vi "UI-电源头正面标签3检测.vi"(8 "error in (no error)":errorcluster caption="错误输入（无错误）", 11 "名称或相对路径":string="Template Program") -> (0 "error in (no error) 2":errorcluster caption="错误输入（无错误）")   [LabVIEW 2017]
uses:
  Global System.vi
  <vilib>/Utility/xml.llb/Write to XML File(string).vi
  Picture/SaveButtom.ctl
panel:
  in  "获取图像":bool
  in  "ROI获取":bool
  in  "创建模板":bool
  in  "保存图像":bool
  out "添加的路径":path
  in  "刷新":bool
  in  "测试按钮":bool
  in  "保存按钮":bool
  in  "Main":enum32{"主参数", "模板匹配参数 ", "测试效果"}(tab)
  in  "UI电源线正面标签3基础参数":T1={"IsNorImage"=TRUE, "Exposure Values"=100289, "ImagePath"=path "C:/Users/hedongpo/Desktop/514-hdp/Alignment Assemble System/Test Picture/B/3.bmp"} caption="参数界面" {"Exposure Values" scale=0.0..200000.0}
  in  "UI电源线正面标签3参数":T3={"Rectangle"={"Left"=0, "Top"=0, "Right"=0, "Bottom"=0, "Rotation"=0.0}, "Algorithm "=2, "Parameters"={"Number of Matches Requested"=1, "Minimum Match Score"=800.0, "Angle Ranges"=[{"Start Angle"=-180.0, "End Angle"=180.0}]}, "Advanced Options "=[{"Item"=102, "Value"=10.0}, {"Item"=106, "Value"=300.0}, {"Item"=107, "Value"=0.0}, {"Item"=108, "Value"=6.0}, {"Item"=109, "Value"=1.0}, {"Item"=114, "Value"=25.0}, {"Item"=111, "Value"=20.0}, {"Item"=112, "Value"=10.0}, {"Item"=113, "Value"=20.0}, {"Item"=103, "Value"=1.0}, {"Item"=104, "Value"=20.0}, {"Item"=105, "Value"=0.0}, {"Item"=100, "Value"=5.0}], "模板路径"=path "", "Color Plane "=0} {"Color Plane" items=["Red", "Green", "Blue", "Hue", "Saturation", "Luminance", "Value", "Intensity"]; "Advanced Options"."Item" items=["LD Sampling - Minimum Constrast"=0, "LD Sampling - Enable Subpixel Accuracy"=1, "LD Sampling - Search Strategy"=2, "LD Sampling - Subpixel Iterations"=3, "LD Sampling - Subpixel Tolerance"=4, "LD Sampling - Initial Match List Length"=5, "LD Sampling - Match List Reduction Factor"=6, "LD Sampling - Initial Step Size"=7, "LD Sampling - Intermediate Angular Accuracy"=8, "-"=9, "Pyramid - Max Pyramid Level"=100, "Pyramid - Minimum Contrast"=102, "Pyramid - Enable Subpixel Accuracy"=103, "Pyramid - Subpixel Iterations"=104, "Pyramid - Subpixel Tolerance"=105, "Pyramid - Initial Match List Length"=106, "Pyramid - Match List Reduction Factor"=107, "Pyramid - Intermediate Angular Accuracy"=108, "Pyramid - Process Border Matches"=109, "Pyramid - Min Match Separation Distance"=111, "Pyramid - Min Match Separation Angle"=112, "Pyramid - Max Match Overlap"=113, "Pyramid - Max Cache in MB"=114, "Pyramid - Clear Cache"=115, "-"=116, "Enable Defect Map"=200]; "Algorithm" items=["All", "Low Discrepancy Sampling", "Grayscale Value Pyramid", "Gradients Pyramid"]; "Rectangle"."Rotation" format="%.2f"; "Rectangle"."Left" scale=0.0..1024.0; "Rectangle"."Right" scale=0.0..1024.0}
  out "结果":bool
  out "原始图像":T4(plugin-control)
  out "模板图片":T4(plugin-control)
  out "路径输出":path
  in  "Vision Paramter Save Buttom":T5
  out "system time":string
  in  "取消按钮":bool
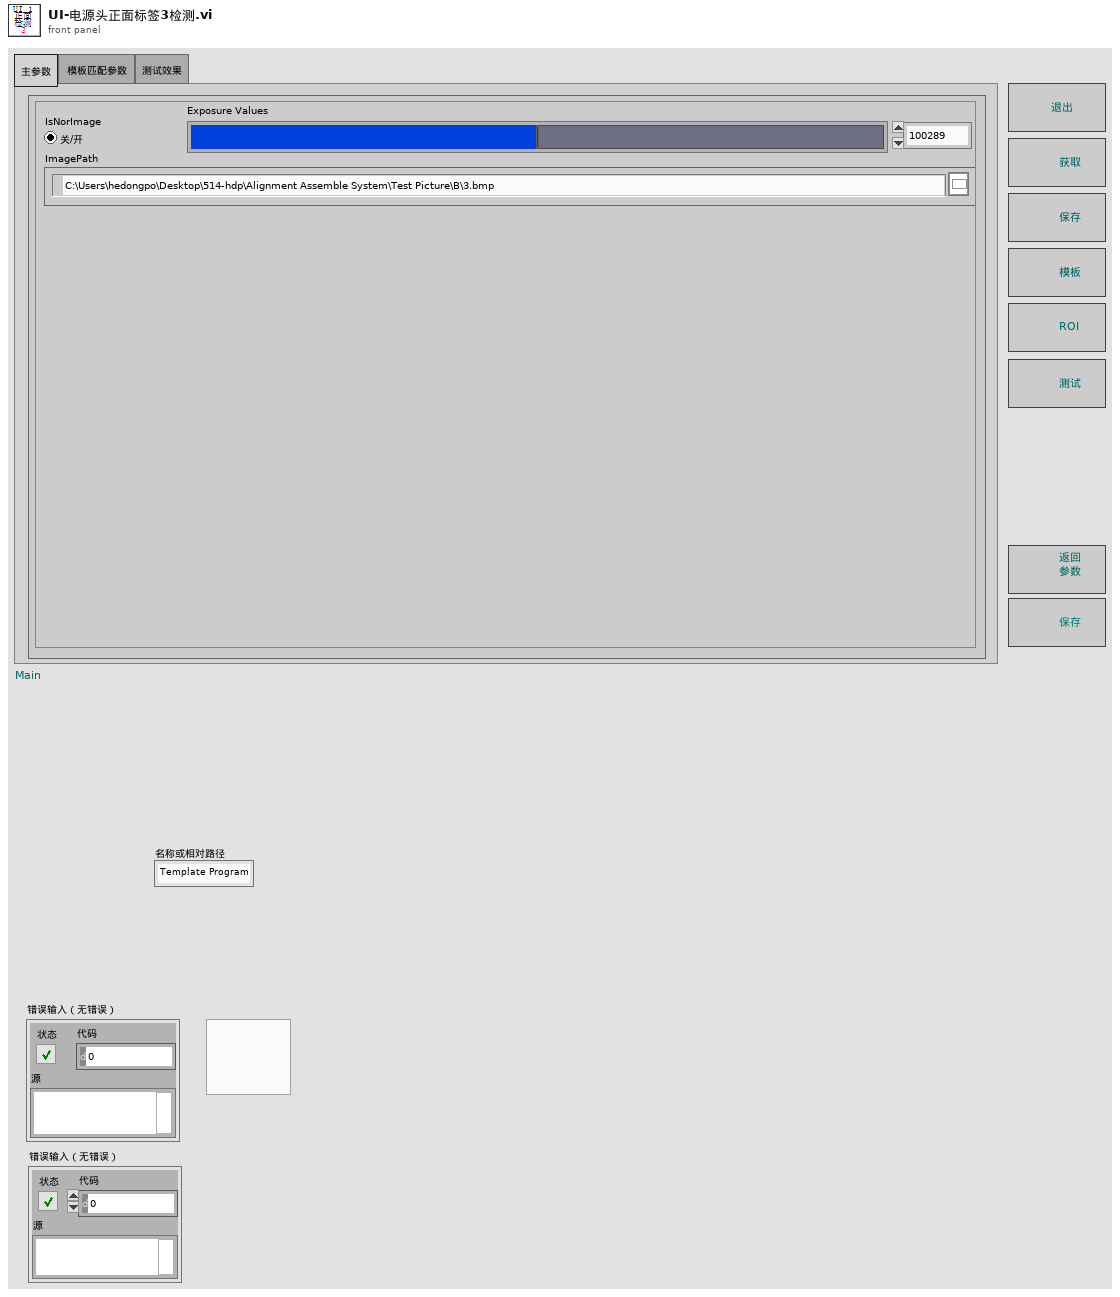
[diagram p1: front panel]
types:
  T1 = cluster{"IsNorImage":bool, "Exposure Values":u32, "ImagePath":path}
  T2 = typedef "IMAQ Rectangle" = cluster{"Left":i32, "Top":i32, "Right":i32, "Bottom":i32, "Rotation":dbl}
  T3 = cluster{"Rectangle":T2, "Algorithm ":i32, "Parameters":cluster{"Number of Matches Requested":i32, "Minimum Match Score":sgl, "Angle Ranges":cluster{"Start Angle":sgl, "End Angle":sgl}[]}, "Advanced Options ":cluster{"Item":u16, "Value":dbl}[], "模板路径":path, "Color Plane ":i32}
  T4 = typedef "IMAQ Image.ctl" = refnum<image>
  T5 = typedef "SaveButtom.ctl" = bool
  T6 = cluster{"index":i32, "this vi":refnum<vi>, "error out":errorcluster}
  T7 = cluster{"master data":string, "priority":u16, "secondary data":string[]}
  T8 = cluster{"case name":string[], "queue array":refnum<queue>[]}
  T9 = typedef "Image Type" = u32
  T10 = cluster{"Global Rectangle":i32[], "Contours":cluster{"Contour Type":u32, "ROI Type":u32, "Points":i32[]}[]}
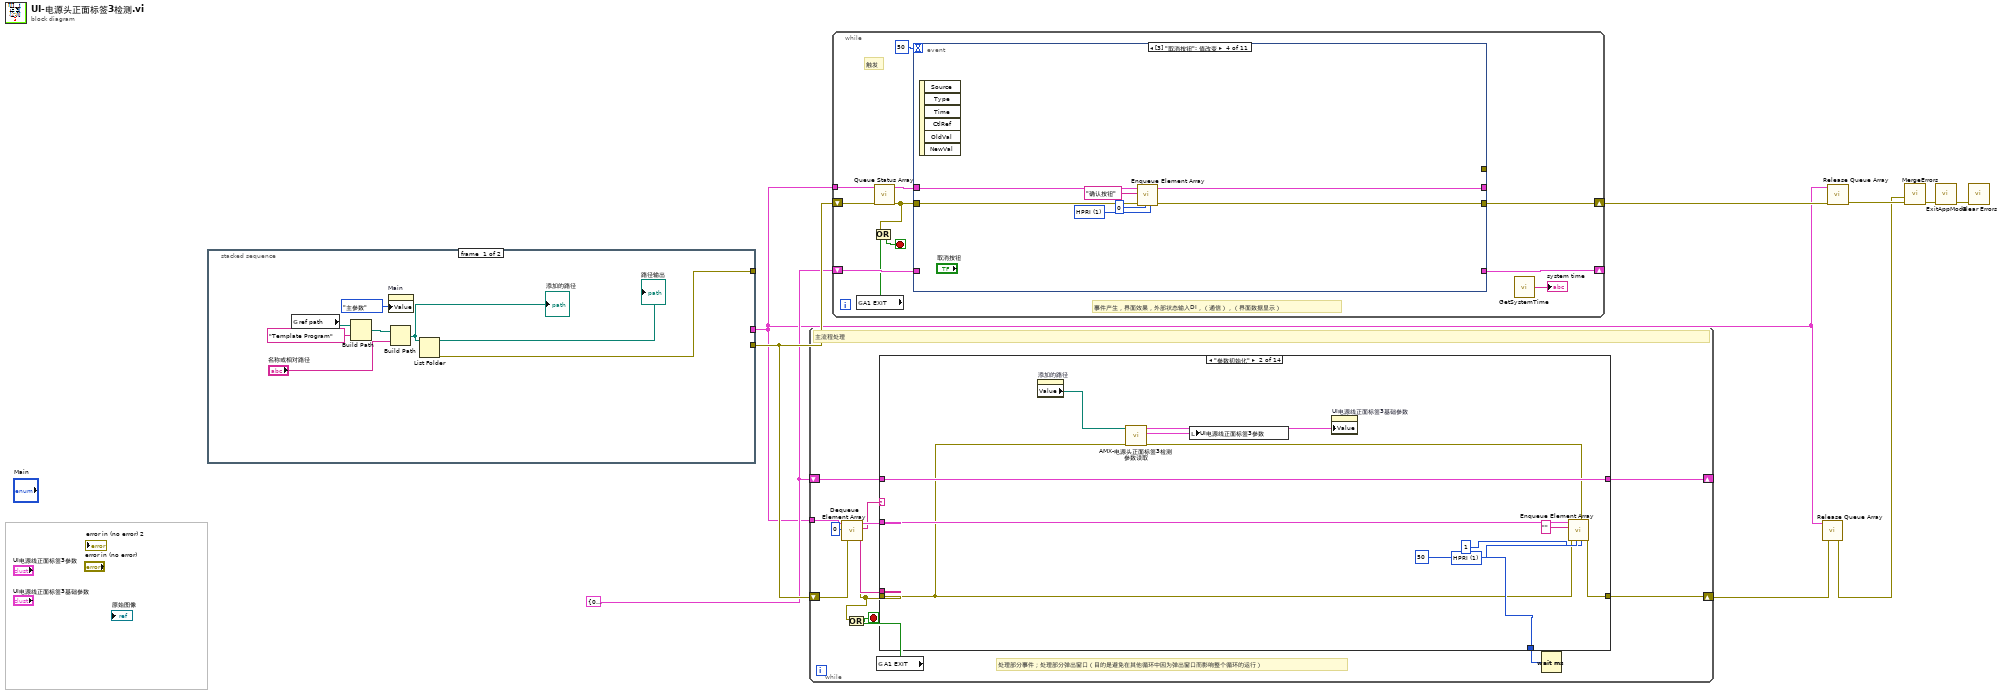
[diagram p0: block diagram]
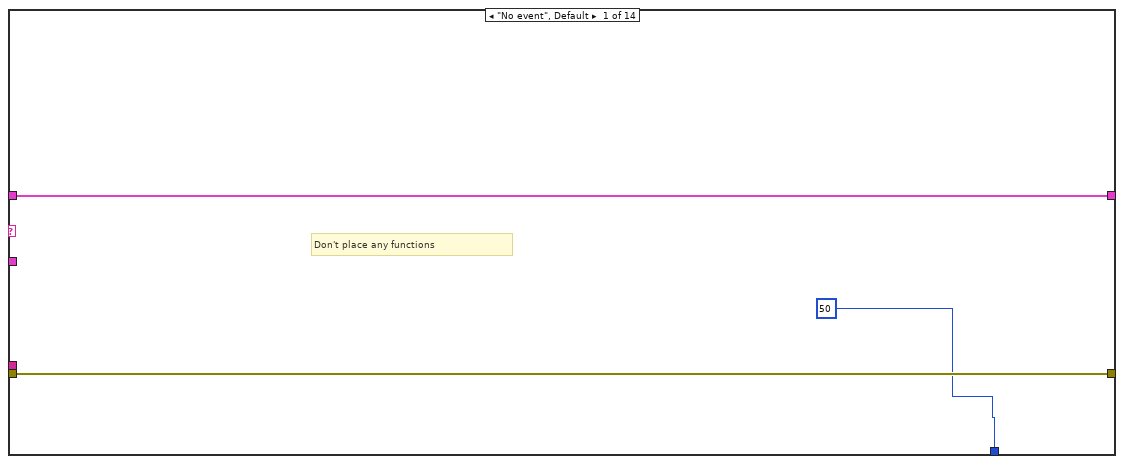
[diagram p2: hidden frame]
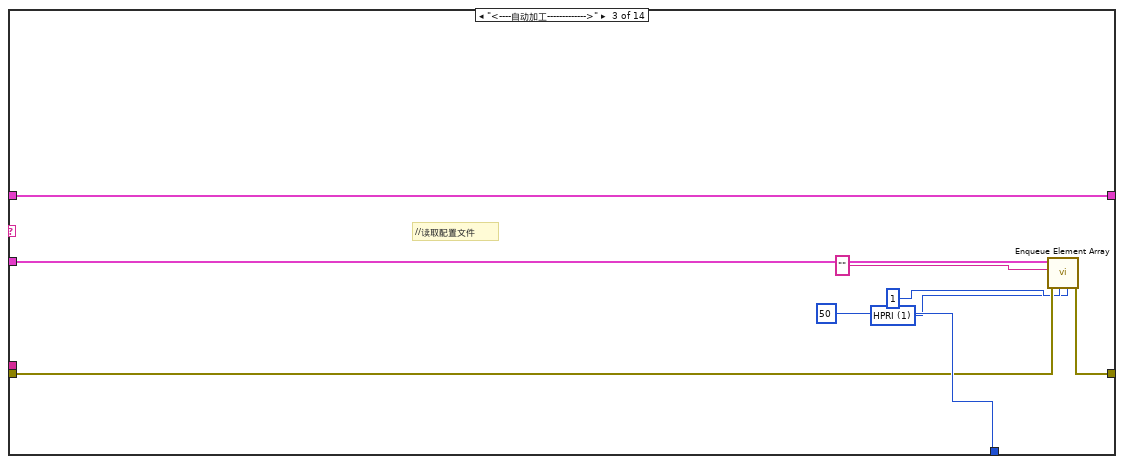
[diagram p3: hidden frame]
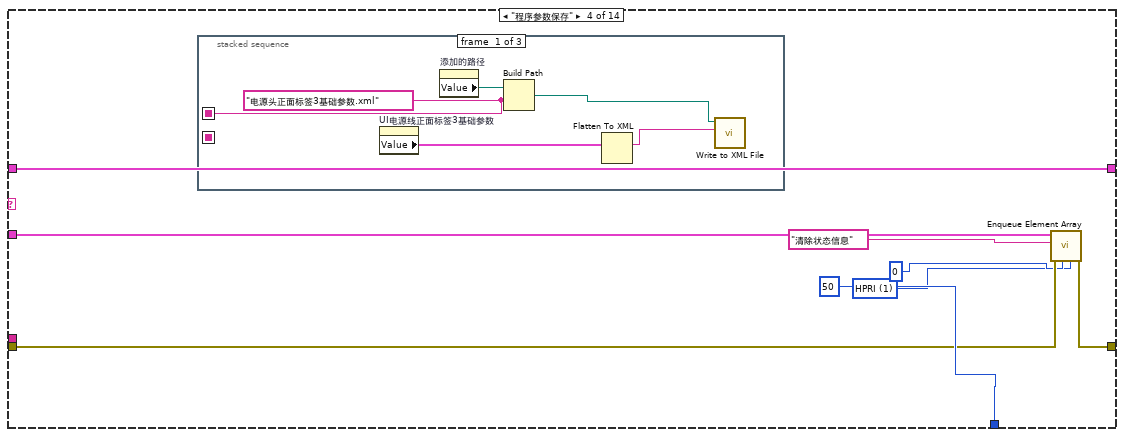
[diagram p4: hidden frame]
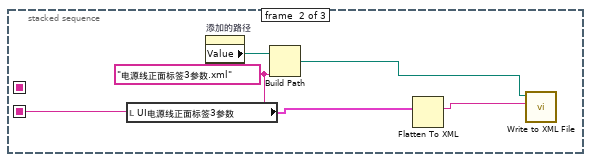
[diagram p5: hidden frame]
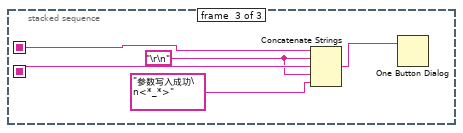
[diagram p6: hidden frame]
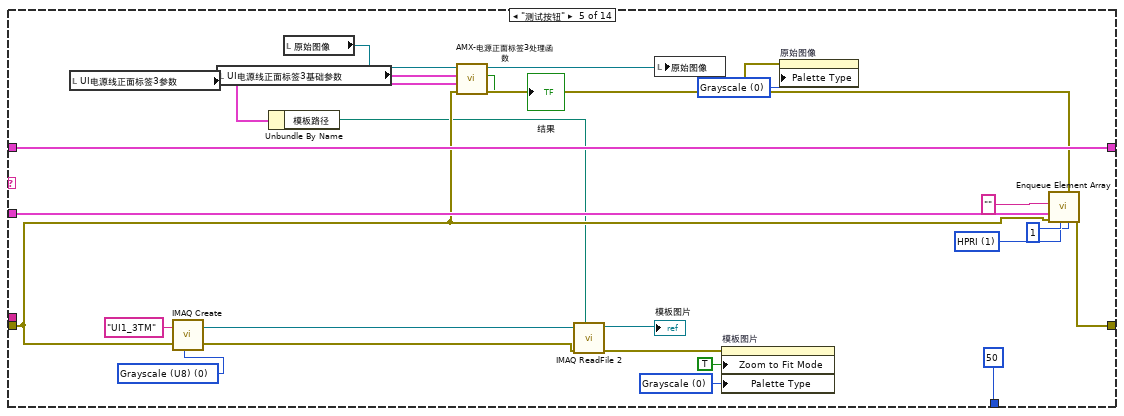
[diagram p7: hidden frame]
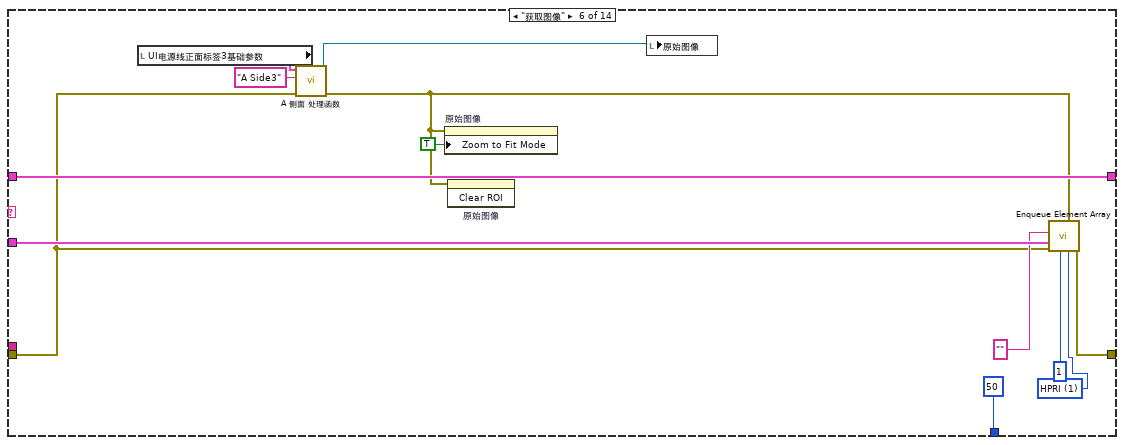
[diagram p8: hidden frame]
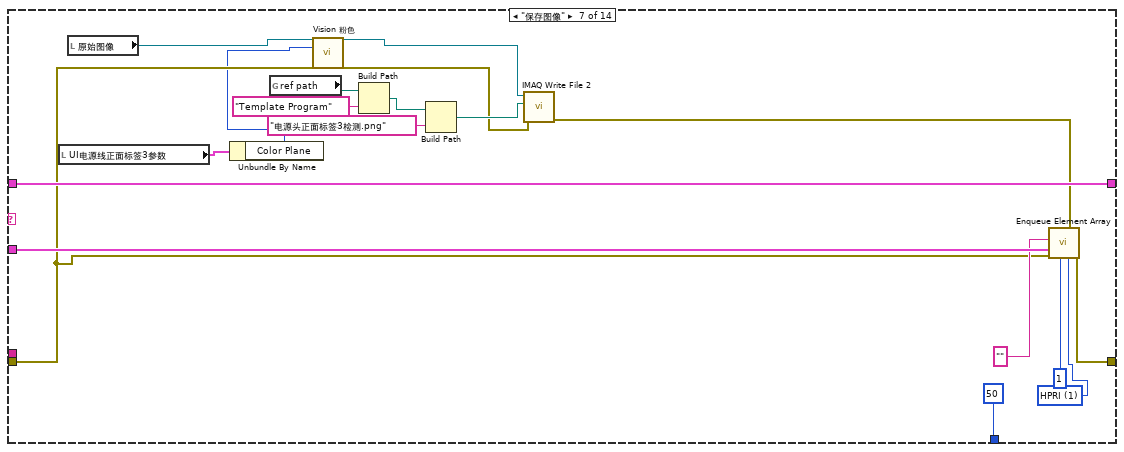
[diagram p9: hidden frame]
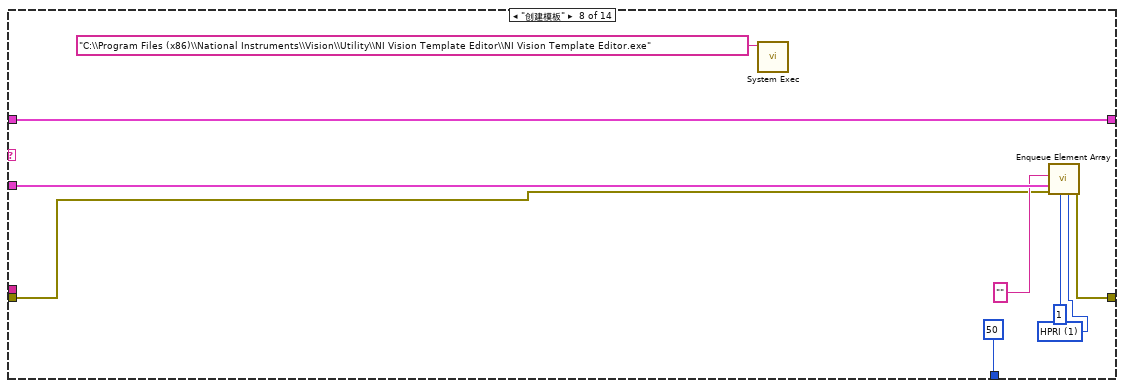
[diagram p10: hidden frame]
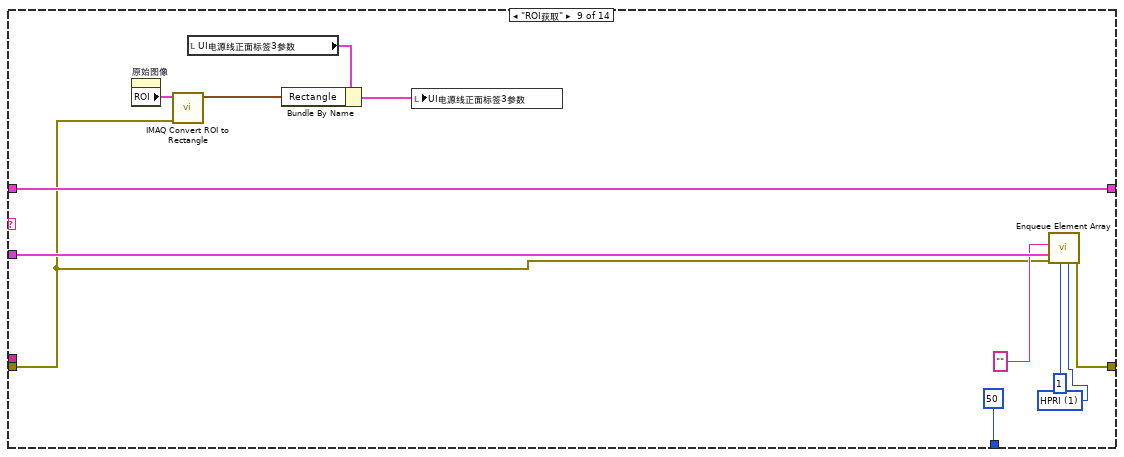
[diagram p11: hidden frame]
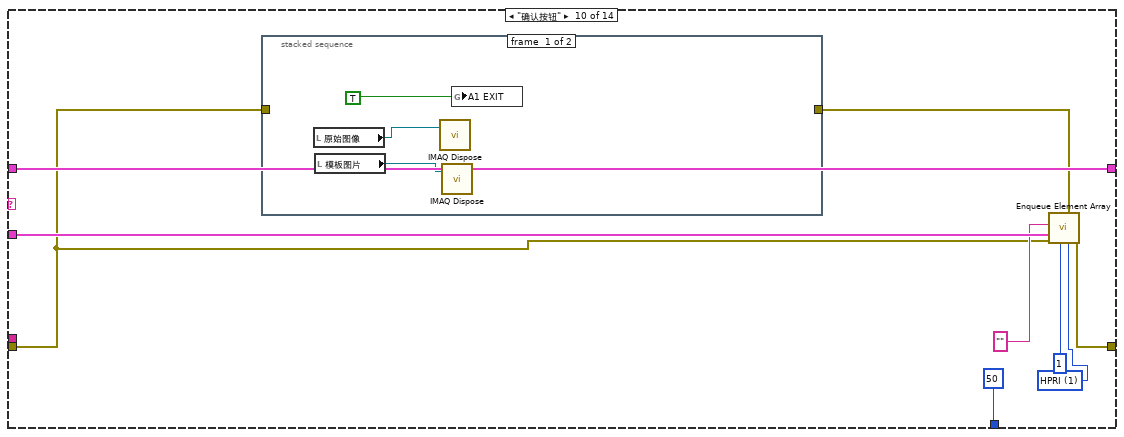
[diagram p12: hidden frame]
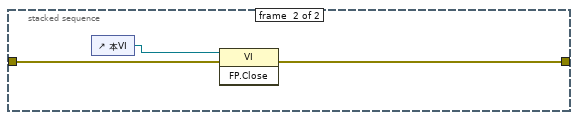
[diagram p13: hidden frame]
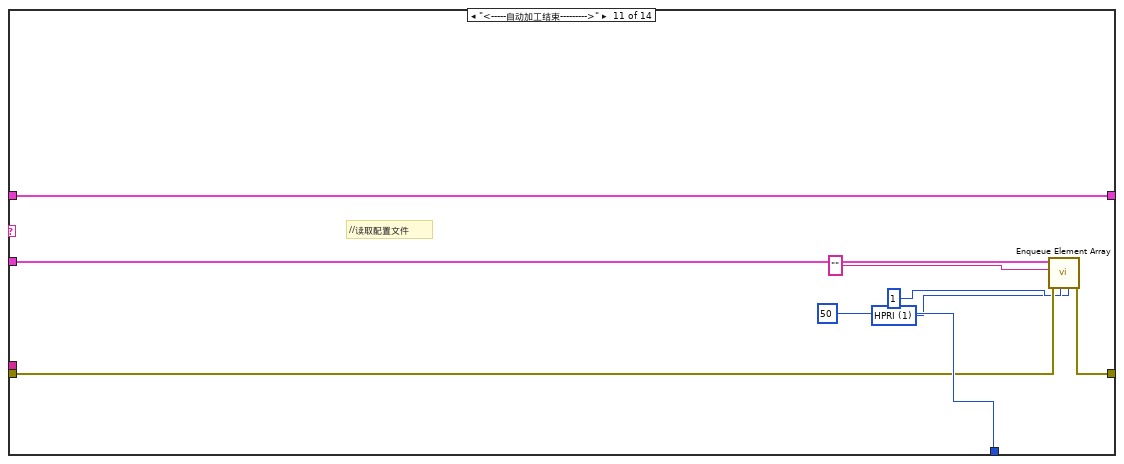
[diagram p14: hidden frame]
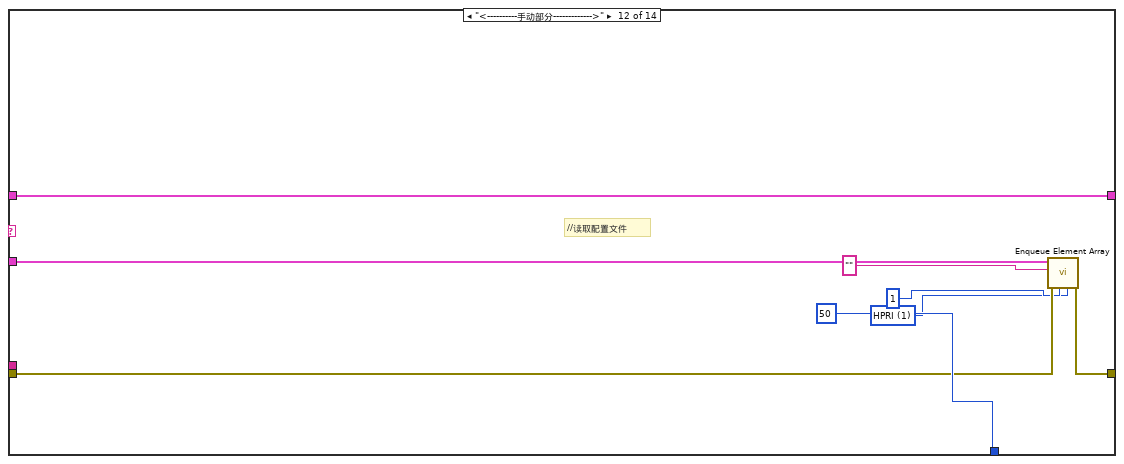
[diagram p15: hidden frame]
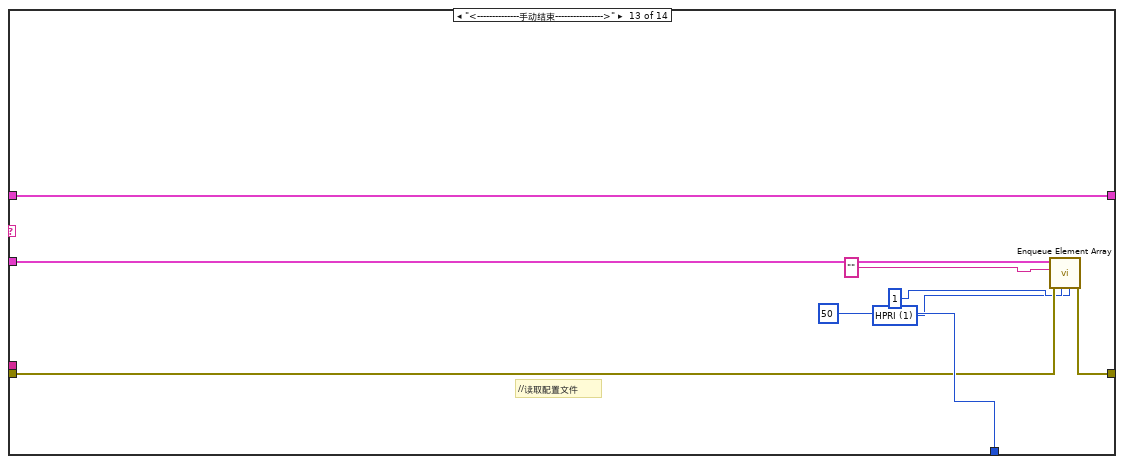
[diagram p16: hidden frame]
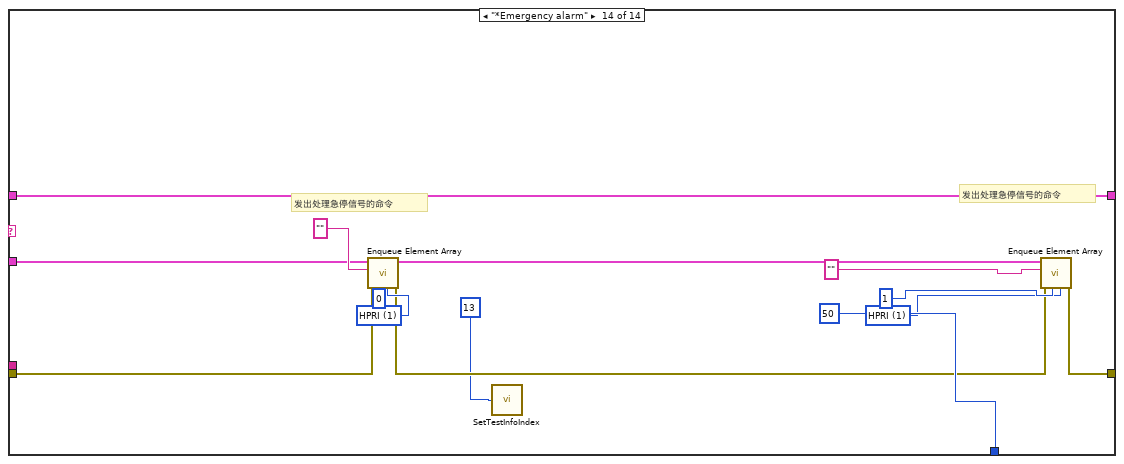
[diagram p17: hidden frame]
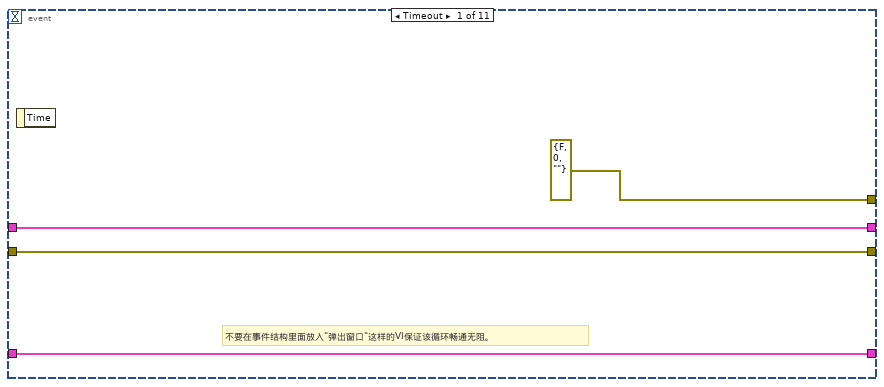
[diagram p18: hidden frame]
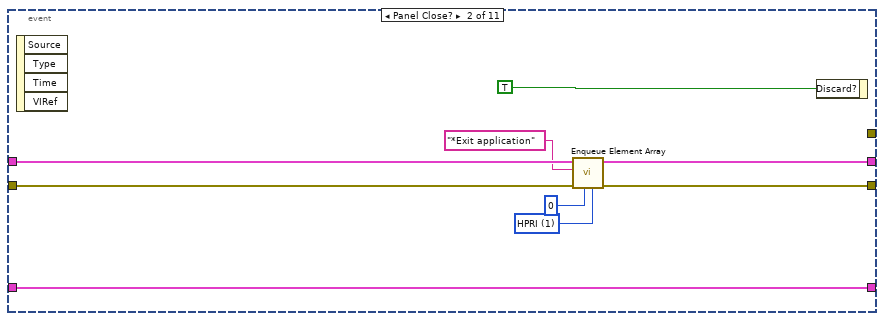
[diagram p19: hidden frame]
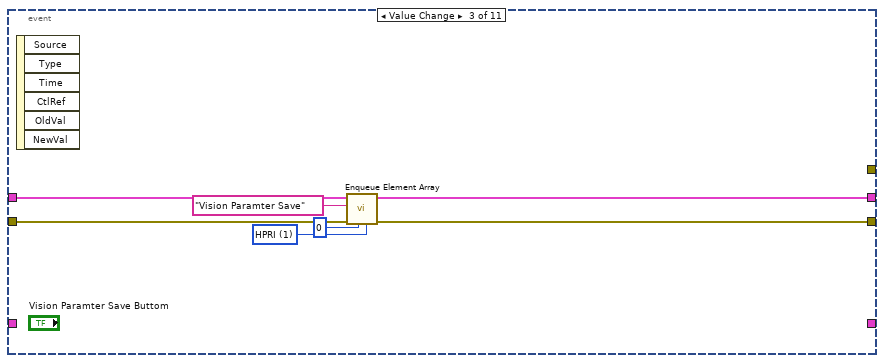
[diagram p20: hidden frame]
diagram:
  w4 = T6 {"index"=0, "this vi"=refnum, "error out"={"status"=FALSE, "code"=0, "source"=""}} ("parameter buffer")
  n1 = stacked-sequence {
    tunnel: [w15 _] -> _
    tunnel: [_ w19] -> w5
    tunnel: [_ w18] -> w1
    frame #0 {
      n2 = global read "Global System.vi" "ref path"() -> (w13:path)
      n3 = Build Path(base path=w13, name or relative path="Template Program" ("名称或相对路径")) -> (appended path=w11:path)
      n4 = property on="Main" class="TabCtl (严格)"("Value"=enum32{"主参数", "模板匹配参数 ", "测试效果"}."主参数" ("Main")) -> ()  [unwired: 2 in, 2 out]
      n5 = Build Path(base path=w11, name or relative path="名称或相对路径") -> (appended path=w17:path)
      "添加的路径" <- w17
      n6 = List Folder(path=w17) -> (path out=→"路径输出":path, error out=w15:errorcluster)  [unwired: 3 in, 2 out]
    }
    frame #1 {
      w27 = string[] ["comm queue1", "data queue 11", "data queue 12", "data queue 13", "data queue 14"]  # queue name
      w28 = 4  # queue num
      w29 = T7 {"master data"="", "priority"=0, "secondary data"=[]}  # element data type
      n7 = call "Obtain Queue Array.vi"("queue name"=w27, "element data type"=w29, "queue num"=w28) -> ("error out"=w23:errorcluster, "queue out"=w24:T8)  [unwired: 2 in, 1 out]
      n8 = call "Enqueue Element Array.vi"("queue index"=0, "error in"=w23, "master data"="参数初始化", "queue in"=w24) -> ("error out"=w22:errorcluster, "queue out"=w21:T8)  [unwired: 6 in]
      n9 = disable-structure shown="启用" {
        disable-tunnel: w22 -> [w35 w36]
        disable-tunnel: w21 -> [w34 w37]
        disable-tunnel: "Loading Variable" ("master data") -> [w33 _]
        disable-tunnel: [w31 w36] -> w19
        disable-tunnel: [w30 w37] -> w18
        frame Disabled {
          n10 = call "Enqueue Element Array.vi"("queue index"=12, "error in"=w35, "master data"=w33, "queue in"=w34) -> ("error out"=w31:errorcluster, "queue out"=w30:T8)  [unwired: 6 in]
        }
        frame Enabled {
        }
      }
    }
  }
  n11 = while {
    shift-right: [w50] -> w3
    shift-left: w5 -> [w41]
    shift-right: [w47] -> _
    shift-left: w4 -> [w48]
    tunnel: w1 -> [w43]
    stop <- w38 stop-if-true
    # "处理部分事件；处理部分弹出窗口（目的是避免在其他循环中因为弹出窗口而影响整个循环的运行）"
    # "主流程处理"
    n12 = call "Dequeue Element Array.vi"("queue in"=w43, "queue index"=0, "error in"=w41) -> ("queue out"=w46:T8, "master data"=w45:string, "secondary data"=w44:string[], "error out"=w40:errorcluster)  [unwired: 2 in, 1 out]
    n13 = global read "Global System.vi" "A1 EXIT"() -> (w39:bool)
    n14 = Or(x=w40, y=w39) -> (x .or. y?=w38:bool)
    n15 = case shown="\"参数初始化\"" w45 {
      tunnel: w46 -> [_ w64 w72 w74 w119 w132 w151 w160 w172 w181 w195 w203 w211 w217]
      tunnel: w40 -> [w52 w57 w68 w78 w112 w123 w137 w154 w165 w175 w191 w199 w207 w214]
      tunnel: [w52 w63 w71 w80 w118 w131 w150 w159 w171 w180 w194 w202 w210 w225] -> w50
      tunnel: [50 50 50 50 50 50 50 50 50 50 50 50 50 50] -> w49
      tunnel: w48 -> [w53 w59 w69 w75 w114 w127 w146 w155 w167 w176 w192 w200 w208 w223]
      tunnel: [w53 w59 w69 w75 w114 w127 w146 w155 w167 w176 w192 w200 w208 w223] -> w47
      tunnel: w44 -> [_ _ _ _ _ _ _ _ _ _ _ _ _ _]
      frame "No event", Default {
        # "Don't place any functions"
      }
      frame "参数初始化" {
        w60 = u16 1 items=["HPRI"=1, "LPRI"=0] ("priority")
        n16 = property on="添加的路径" class="Path"() -> ("Value"=w58:path)  [unwired: 2 in, 2 out]
        n17 = call "AMX-电源头正面标签3检测参数读取.vi"("error in (no error)"=w57, "基路径"=w58) -> ("error out"=w56:errorcluster, "UI电源线正面标签3参数"=w54:T3, "UI电源线正面标签3基础参数"=w55:T1)  [unwired: 6 in]
        n18 = local write "UI电源线正面标签3参数"(w54) -> ()
        n19 = property on="UI电源线正面标签3基础参数" class="Clust (严格)"("Value"=w55) -> ()  [unwired: 2 in, 2 out]
        n20 = call "Enqueue Element Array.vi"("priority"=w60, "device error in"=w56, "queue index"=1, "error in"=w57, "master data"="" ("Element 1"), "queue in"=w64) -> ("error out"=w63:errorcluster)  [unwired: 4 in, 1 out]
      }
      frame "<----自动加工------------->" {
        w66 = u16 1 items=["HPRI"=1, "LPRI"=0] ("priority")
        # "//读取配置文件"
        n21 = call "Enqueue Element Array.vi"("priority"=w66, "queue index"=1, "error in"=w68, "master data"="" ("Element 1"), "queue in"=w72) -> ("error out"=w71:errorcluster)  [unwired: 5 in, 1 out]
      }
      frame "程序参数保存" {
        w76 = u16 1 items=["HPRI"=1, "LPRI"=0] ("priority")
        n22 = stacked-sequence {
          seq-local: [w82 _ _] -> [_ _ w95]
          seq-local: [_ w88 _] -> [_ _ w93]
          frame #0 {
            w82 = "电源头正面标签3基础参数.xml" ("名称或相对路径")
            n23 = property on="UI电源线正面标签3基础参数" class="Clust (严格)"() -> ("Value"=w85:T1)  [unwired: 2 in, 2 out]
            n24 = property on="添加的路径" class="Path"() -> ("Value"=w86:path)  [unwired: 2 in, 2 out]
            n25 = Build Path(base path=w86, name or relative path=w82) -> (appended path=w83:path)
            n26 = Flatten To XML(anything=w85) -> (xml string=w84:string)
            n27 = call-poly <vilib>:"Write to XML File.vi"("XML Input"=w84, "XML File Path"=w83) -> ()  [unwired: 7 in, 3 out]
          }
          frame #1 {
            w88 = "电源线正面标签3参数.xml" ("名称或相对路径")
            n28 = local read "UI电源线正面标签3参数"() -> (w87:T3)
            n29 = property on="添加的路径" class="Path"() -> ("Value"=w91:path)  [unwired: 2 in, 2 out]
            n30 = Build Path(base path=w91, name or relative path=w88) -> (appended path=w89:path)
            n31 = Flatten To XML(anything=w87) -> (xml string=w90:string)
            n32 = call-poly <vilib>:"Write to XML File.vi"("XML Input"=w90, "XML File Path"=w89) -> ()  [unwired: 7 in, 3 out]
          }
          frame #2 {
            w92 = "\r\n"
            n33 = Concatenate Strings(w95, w92, w93, w92, "参数写入成功\n<*_*>" ("消息")) -> (w94:string)
            n34 = One Button Dialog(message=w94) -> ()  [unwired: 1 in, 1 out]
          }
        }
        n35 = call "Enqueue Element Array.vi"("priority"=w76, "queue index"=0, "error in"=w78, "master data"="清除状态信息" ("Element 1"), "queue in"=w74) -> ("error out"=w80:errorcluster)  [unwired: 5 in, 1 out]
      }
      frame "测试按钮" {
        w99 = u32 0 items=["Grayscale", "Binary", "Gradient", "Rainbow", "Temperature", "User Defined", "Binary 16 Bit", "Gradient 16 Bit", "Rainbow 16 Bit", "Temperature 16 Bit", "User Defined 16 Bit"] ("Palette:Palette Type")
        w105 = T9 0 items=["Grayscale (U8)", "Grayscale (I16)", "Grayscale (SGL)", "Complex (CSG)", "RGB (U32)", "HSL (U32)", "RGB (U64)", "Grayscale (U16)"] ("Image Type")
        w107 = u32 0 items=["Grayscale", "Binary", "Gradient", "Rainbow", "Temperature", "User Defined", "Binary 16 Bit", "Gradient 16 Bit", "Rainbow 16 Bit", "Temperature 16 Bit", "User Defined 16 Bit"] ("Palette:Palette Type")
        w115 = u16 1 items=["HPRI"=1, "LPRI"=0] ("priority")
        n36 = local read "UI电源线正面标签3参数"() -> (w110:T3)
        n37 = call "IMAQ Create"("Image Name"="UI1_3TM", "Image Type"=w105, "error in (no error)"=w112) -> ("New Image"=w104:T4, "error out"=w103:errorcluster)  [unwired: 2 in]
        n38 = local read "UI电源线正面标签3基础参数"() -> (w113:T1)
        n39 = Unbundle By Name(w110) -> ("模板路径"=w98:path)
        n40 = local read "原始图像"() -> (w109:T4)
        n41 = call "AMX-电源正面标签3处理函数.vi"("error in (no error)"=w112, "UI电源线正面标签1参数"=w110, "电源线正面标签1基础参数"=w113, "Image in"=w109) -> ("error out"=w108:errorcluster, "j结果"=→"结果":bool, "Image out"=w111:T4)  [unwired: 4 in, 1 out]
        n42 = call "IMAQ ReadFile 2"("File Path"=w98, "error in (no error)"=w103, "Image"=w104) -> ("error out"=w101:errorcluster, "Image Out"=→"模板图片":T4)  [unwired: 4 in, 3 out]
        n43 = local write "原始图像"(w111) -> ()
        n44 = property on="模板图片" class="ImageControl"(error in=w101, "Zoom to Fit Mode"=TRUE, "Palette Type"=w99) -> ()  [unwired: 1 in, 2 out]
        n45 = property on="原始图像" class="ImageControl"(error in=w108, "Palette Type"=w107) -> ()  [unwired: 1 in, 2 out]
        n46 = call "Enqueue Element Array.vi"("priority"=w115, "device error in"=w108, "queue index"=1, "error in"=w112, "master data"="" ("Element 1"), "queue in"=w119) -> ("error out"=w118:errorcluster)  [unwired: 4 in, 1 out]
      }
      frame "获取图像" {
        w128 = u16 1 items=["HPRI"=1, "LPRI"=0] ("priority")
        n47 = local read "UI电源线正面标签3基础参数"() -> (w125:T1)
        n48 = call "A 侧面 处理函数.vi"("error in (no error)"=w123, "Image Name"="A Side3", "ParamsUI"=w125) -> ("error out"=w121:errorcluster, "Image out"=w124:T4)  [unwired: 5 in, 2 out]
        n49 = property on="原始图像" class="ImageControl"(error in=w121, "Zoom to Fit Mode"=TRUE) -> ()  [unwired: 1 in, 2 out]
        n50 = invoke on="原始图像" class="ImageControl" method="Clear ROI"(error in=w121) -> ()  [unwired: 2 in, 3 out]
        n51 = local write "原始图像"(w124) -> ()
        n52 = call "Enqueue Element Array.vi"("priority"=w128, "device error in"=w121, "queue index"=1, "error in"=w123, "master data"="" ("Element 1"), "queue in"=w132) -> ("error out"=w131:errorcluster)  [unwired: 4 in, 1 out]
      }
      frame "保存图像" {
        w147 = u16 1 items=["HPRI"=1, "LPRI"=0] ("priority")
        n53 = local read "UI电源线正面标签3参数"() -> (w135:T3)
        n54 = local read "原始图像"() -> (w139:T4)
        n55 = Unbundle By Name(w135) -> ("Color Plane"=w134:i32)
        n56 = global read "Global System.vi" "ref path"() -> (w145:path)
        n57 = call "Vision 粉色"("Image In"=w139, "Color Plane (Color Plane Extraction 1)"=w134, "error in"=w137) -> ("Image Out"=w138:T4, "error out"=w136:errorcluster)  [unwired: 23 in]
        n58 = Build Path(base path=w145, name or relative path="Template Program" ("名称或相对路径")) -> (appended path=w143:path)
        n59 = Build Path(base path=w143, name or relative path="电源头正面标签3检测.png" ("名称或相对路径")) -> (appended path=w141:path)
        n60 = call-poly "IMAQ Write File 2"("error in (no error)"=w136, "File Path"=w141, "Image"=w138) -> ("error out"=w140:errorcluster)  [unwired: 7 in, 1 out]
        n61 = call "Enqueue Element Array.vi"("priority"=w147, "device error in"=w140, "queue index"=1, "error in"=w137, "master data"="" ("Element 1"), "queue in"=w151) -> ("error out"=w150:errorcluster)  [unwired: 4 in, 1 out]
      }
      frame "创建模板" {
        w156 = u16 1 items=["HPRI"=1, "LPRI"=0] ("priority")
        n62 = call <vilib>:"System Exec.vi"("command line"="C:\\Program Files (x86)\\National Instruments\\Vision\\Utility\\NI Vision Template Editor\\NI Vision Template Editor.exe") -> ()  [unwired: 7 in, 4 out]
        n63 = call "Enqueue Element Array.vi"("priority"=w156, "queue index"=1, "error in"=w154, "master data"="" ("Element 1"), "queue in"=w160) -> ("error out"=w159:errorcluster)  [unwired: 5 in, 1 out]
      }
      frame "ROI获取" {
        w168 = u16 1 items=["HPRI"=1, "LPRI"=0] ("priority")
        n64 = property on="原始图像" class="ImageControl"() -> ("ROI"=w166:T10)  [unwired: 2 in, 2 out]
        n65 = call "IMAQ Convert ROI to Rectangle"("error in (no error)"=w165, "ROI Descriptor"=w166) -> ("Rectangle"=w163:T2)  [unwired: 7 in, 1 out]
        n66 = local read "UI电源线正面标签3参数"() -> (w164:T3)
        n67 = Bundle By Name(cluster=w164, "Rectangle"=w163) -> (w162:T3)
        n68 = local write "UI电源线正面标签3参数"(w162) -> ()
        n69 = call "Enqueue Element Array.vi"("priority"=w168, "queue index"=1, "error in"=w165, "master data"="" ("Element 1"), "queue in"=w172) -> ("error out"=w171:errorcluster)  [unwired: 5 in, 1 out]
      }
      frame "确认按钮" {
        w177 = u16 1 items=["HPRI"=1, "LPRI"=0] ("priority")
        n70 = stacked-sequence {
          tunnel: w175 -> [_ w187]
          tunnel: [_ w186] -> w174
          frame #0 {
            n71 = local read "原始图像"() -> (w184:T4)
            n72 = local read "模板图片"() -> (w183:T4)
            n73 = call "IMAQ Dispose"("Image"=w184) -> ()  [unwired: 5 in, 1 out]
            n74 = call "IMAQ Dispose"("Image"=w183) -> ()  [unwired: 5 in, 1 out]
            n75 = global write "Global System.vi" "A1 EXIT"(TRUE ("EXIT")) -> ()
          }
          frame #1 {
            n76 = control-ref of="本VI"() -> (w188:refnum<vi>)
            n77 = invoke class="VI" method="FP.Close"(reference=w188, error in=w187) -> (error out=w186:errorcluster)  [unwired: 1 in, 2 out]
          }
        }
        n78 = call "Enqueue Element Array.vi"("priority"=w177, "device error in"=w174, "queue index"=1, "error in"=w175, "master data"="" ("Element 1"), "queue in"=w181) -> ("error out"=w180:errorcluster)  [unwired: 4 in, 1 out]
      }
      frame "<-----自动加工结束--------->" {
        w189 = u16 1 items=["HPRI"=1, "LPRI"=0] ("priority")
        # "//读取配置文件"
        n79 = call "Enqueue Element Array.vi"("priority"=w189, "queue index"=1, "error in"=w191, "master data"="" ("Element 1"), "queue in"=w195) -> ("error out"=w194:errorcluster)  [unwired: 5 in, 1 out]
      }
      frame "<----------手动部分------------->" {
        w197 = u16 1 items=["HPRI"=1, "LPRI"=0] ("priority")
        # "//读取配置文件"
        n80 = call "Enqueue Element Array.vi"("priority"=w197, "queue index"=1, "error in"=w199, "master data"="" ("Element 1"), "queue in"=w203) -> ("error out"=w202:errorcluster)  [unwired: 5 in, 1 out]
      }
      frame "<--------------手动结束---------------->" {
        w205 = u16 1 items=["HPRI"=1, "LPRI"=0] ("priority")
        # "//读取配置文件"
        n81 = call "Enqueue Element Array.vi"("priority"=w205, "queue index"=1, "error in"=w207, "master data"="" ("Element 1"), "queue in"=w211) -> ("error out"=w210:errorcluster)  [unwired: 5 in, 1 out]
      }
      frame "*Emergency alarm" {
        w220 = u16 1 items=["HPRI"=1, "LPRI"=0] ("priority")
        w221 = u16 1 items=["HPRI"=1, "LPRI"=0] ("priority")
        # "发出处理急停信号的命令"
        # "发出处理急停信号的命令"
        n82 = call "Enqueue Element Array.vi"("priority"=w220, "queue index"=0, "error in"=w214, "master data"="" ("Element 1"), "queue in"=w217) -> ("error out"=w215:errorcluster, "queue out"=w216:T8)  [unwired: 5 in]
        n83 = call "SetTestInfoIndex.vi"("test info index"=13) -> ()
        n84 = call "Enqueue Element Array.vi"("priority"=w221, "queue index"=1, "error in"=w215, "master data"="" ("Element 1"), "queue in"=w216) -> ("error out"=w225:errorcluster)  [unwired: 5 in, 1 out]
      }
    }
    n85 = Wait (ms)(milliseconds to wait=w49) -> ()  [unwired: 1 out]
  }
  n86 = while {
    shift-right: [w230] -> w6
    shift-left: w5 -> [w234]
    shift-right: [w232] -> _
    shift-left: w4 -> [w233]
    tunnel: w1 -> [w236]
    stop <- w227 stop-if-true
    # "触发"
    # "事件产生，界面效果，外部状态输入DI，（通信），（界面数据显示）"
    n87 = global read "Global System.vi" "A1 EXIT"() -> (w228:bool)
    n88 = call "Queue Status Array.vi"("error in (no error)"=w234, "queue in"=w236) -> ("error out"=w229:errorcluster, "queue out"=w231:T8)  [unwired: 4 in]
    n89 = Or(x=w229, y=w228) -> (x .or. y?=w227:bool)
    n90 = event shown="[3] \"取消按钮\": 值改变" {
      selector: _ -> [_ _ _ _ _ _ _ _ _ _ _]
      dyn-events: _ -> [_ _ _ _ _ _ _ _ _ _ _]
      timeout: 50 -> [_ _ _ _ _ _ _ _ _ _ _]
      tunnel: w233 -> [w241 w249 _ _ _ _ _ _ _ _ _]
      tunnel: [w241 w249 _ _ _ _ _ _ _ _ _] -> w232
      tunnel: [errorcluster {"status"=FALSE, "code"=0, "source"=""} ("error out") _ _ _ _ _ _ _ _ _ _] -> _
      tunnel: w231 -> [w239 w248 w254 w261 w268 w276 w283 w290 w298 w306 w314]
      tunnel: w229 -> [w238 w247 w253 w260 w267 w275 w282 w289 w297 w305 w313]
      tunnel: [w238 w246 w251 w258 w265 w273 w280 w287 w295 w303 w311] -> w230
      tunnel: [w239 w245 w252 w259 w266 w274 w281 w288 w296 w304 w312] -> _
      event Timeout {
        # "不要在事件结构里面放入\"弹出窗口\"这样的VI保证该循环畅通无阻。"
        n91 = event-data() -> ()  [unwired: 1 in, 1 out]
      }
      event Panel Close? {
        w243 = u16 1 items=["HPRI"=1, "LPRI"=0] ("priority")
        n92 = event-data() -> ()  [unwired: 1 in, 4 out]
        n93 = call "Enqueue Element Array.vi"("priority"=w243, "queue index"=0, "error in"=w247, "master data"="*Exit application", "queue in"=w248) -> ("error out"=w246:errorcluster, "queue out"=w245:T8)  [unwired: 5 in]
        n94 = event-data("Discard?"=TRUE) -> ()  [unwired: 1 in, 1 out]
      }
      event Value Change {
        w256 = u16 1 items=["HPRI"=1, "LPRI"=0] ("priority")
        n95 = event-data() -> ()  [unwired: 1 in, 6 out]
        n96 = call "Enqueue Element Array.vi"("priority"=w256, "queue index"=0, "error in"=w253, "master data"="Vision Paramter Save", "queue in"=w254) -> ("error out"=w251:errorcluster, "queue out"=w252:T8)  [unwired: 5 in]
      }
      event "取消按钮": Value Change {
        w263 = u16 1 items=["HPRI"=1, "LPRI"=0] ("priority")
        n97 = event-data() -> ()  [unwired: 1 in, 6 out]
        n98 = call "Enqueue Element Array.vi"("priority"=w263, "queue index"=0, "error in"=w260, "master data"="确认按钮", "queue in"=w261) -> ("error out"=w258:errorcluster, "queue out"=w259:T8)  [unwired: 5 in]
      }
      event "保存按钮": Value Change {
        w270 = u16 1 items=["HPRI"=1, "LPRI"=0] ("priority")
        n99 = event-data() -> ()  [unwired: 1 in, 6 out]
        n100 = call "Enqueue Element Array.vi"("priority"=w270, "queue index"=0, "error in"=w267, "master data"="程序参数保存", "queue in"=w268) -> ("error out"=w265:errorcluster, "queue out"=w266:T8)  [unwired: 5 in]
      }
      event "获取图像": Value Change {
        w278 = u16 1 items=["HPRI"=1, "LPRI"=0] ("priority")
        n101 = event-data() -> ()  [unwired: 1 in, 6 out]
        n102 = property on="Main" class="TabCtl (严格)"("Value"=enum32{"主参数", "模板匹配参数 ", "测试效果"}."测试效果" ("Main")) -> ()  [unwired: 2 in, 2 out]
        n103 = call "Enqueue Element Array.vi"("priority"=w278, "queue index"=0, "error in"=w275, "master data"="获取图像", "queue in"=w276) -> ("error out"=w273:errorcluster, "queue out"=w274:T8)  [unwired: 5 in]
      }
      event "保存图像": Value Change {
        w285 = u16 1 items=["HPRI"=1, "LPRI"=0] ("priority")
        n104 = event-data() -> ()  [unwired: 1 in, 6 out]
        n105 = call "Enqueue Element Array.vi"("priority"=w285, "queue index"=0, "error in"=w282, "master data"="保存图像", "queue in"=w283) -> ("error out"=w280:errorcluster, "queue out"=w281:T8)  [unwired: 5 in]
      }
      event "创建模板": Value Change {
        w292 = u16 1 items=["HPRI"=1, "LPRI"=0] ("priority")
        n106 = event-data() -> ()  [unwired: 1 in, 6 out]
        n107 = call "Enqueue Element Array.vi"("priority"=w292, "queue index"=0, "error in"=w289, "master data"="创建模板", "queue in"=w290) -> ("error out"=w287:errorcluster, "queue out"=w288:T8)  [unwired: 5 in]
      }
      event "ROI获取": Value Change {
        w300 = u16 1 items=["HPRI"=1, "LPRI"=0] ("priority")
        n108 = event-data() -> ()  [unwired: 1 in, 6 out]
        n109 = property on="Main" class="TabCtl (严格)"("Value"=enum32{"主参数", "模板匹配参数 ", "测试效果"}."模板匹配参数 " ("Main")) -> ()  [unwired: 2 in, 2 out]
        n110 = call "Enqueue Element Array.vi"("priority"=w300, "queue index"=0, "error in"=w297, "master data"="ROI获取", "queue in"=w298) -> ("error out"=w295:errorcluster, "queue out"=w296:T8)  [unwired: 5 in]
      }
      event "测试按钮": Value Change {
        w308 = u16 1 items=["HPRI"=1, "LPRI"=0] ("priority")
        n111 = event-data() -> ()  [unwired: 1 in, 6 out]
        n112 = property on="Main" class="TabCtl (严格)"("Value"=enum32{"主参数", "模板匹配参数 ", "测试效果"}."测试效果" ("Main")) -> ()  [unwired: 2 in, 2 out]
        n113 = call "Enqueue Element Array.vi"("priority"=w308, "queue index"=0, "error in"=w305, "master data"="测试按钮", "queue in"=w306) -> ("error out"=w303:errorcluster, "queue out"=w304:T8)  [unwired: 5 in]
      }
      event "刷新": Value Change {
        n114 = event-data() -> ()  [unwired: 1 in, 6 out]
        n115 = disable-structure shown="禁用" {
          disable-tunnel: w314 -> [w318 _]
          disable-tunnel: w313 -> [w317 _]
          disable-tunnel: [w316 _] -> w312
          disable-tunnel: [w315 _] -> w311
          frame Disabled {
            w320 = u16 1 items=["HPRI"=1, "LPRI"=0] ("priority")
            # "刷新"
            n116 = call "Enqueue Element Array.vi"("priority"=w320, "queue index"=0, "error in"=w317, "master data"="刷新", "queue in"=w318) -> ("error out"=w315:errorcluster, "queue out"=w316:T8)  [unwired: 5 in]
          }
          frame Enabled {
          }
        }
        n117 = property on="Main" class="TabCtl (严格)"("Value"=enum32{"主参数", "模板匹配参数 ", "测试效果"}."模板匹配参数 " ("Main")) -> ()  [unwired: 2 in, 2 out]
      }
    }
    n118 = call "GetSystemTime.vi"() -> ("date/time string"=→"system time":string)  [unwired: 7 in]
  }
  n119 = call "Release Queue Array.vi"("error in"=w3, "queue in"=w1) -> ("error out"=w2:errorcluster)  [unwired: 2 in, 3 out]
  n120 = call "Release Queue Array.vi"("error in"=w6, "queue in"=w1) -> ("error out"=w9:errorcluster)  [unwired: 2 in, 3 out]
  n121 = call "MergeErrors.vi"("error in 3 (no error)"=w2, "error in 4 (no error)"=w9) -> ("error out"=w8:errorcluster)  [unwired: 6 in]
  n122 = call "ExitAppMode.vi"("error in (no error)"=w8) -> ("error out"=w7:errorcluster)  [unwired: 10 in]
  n123 = call <vilib>:"Clear Errors.vi"("error in (no error)"=w7) -> ()  [unwired: 5 in, 2 out]
